vi "To Serial Form.vi"(6 "Serial Version":T1, 10 "Serializer in":refnum<class "Serializer.lvclass">=refnum, 11 "AlicatCommBank in":refnum<class "AlicatCommBank.lvclass">=refnum) -> (0 "error out":errorcluster, 2 "Serializer out":refnum<class "Serializer.lvclass">, 3 "AlicatCommBank out":refnum<class "AlicatCommBank.lvclass">)   [LabVIEW 2014]
uses:
  <userlib>/Serialization/Serializable/Insert Serializable.vi
  <userlib>/Serialization/Serializer/Serializer.lvclass
  <userlib>/Serialization/Serialization Common/Serial Version.ctl
  AlicatCommBank.lvclass
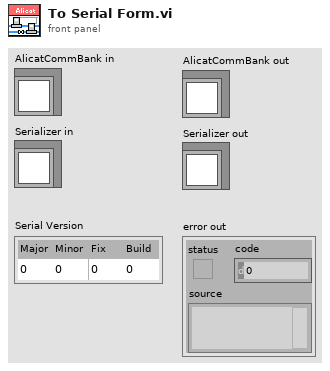
[diagram p1: front panel]
types:
  T1 = typedef "Serialization Common.lvlib/Serial Version.ctl" = cluster{"Major":u16, "Minor":u16, "Fix":u16, "Build":u16}
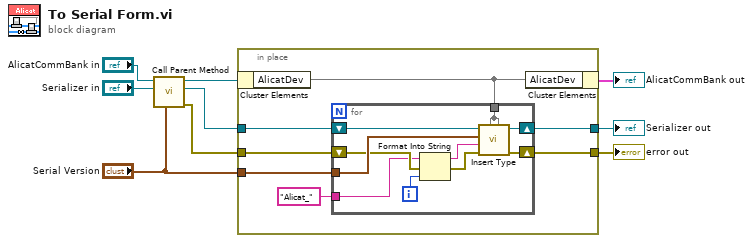
[diagram p0: block diagram]
diagram:
  n1 = call-parent "Call Parent Method"("Serial Version"="Serial Version", "Serializer in"="Serializer in", "Serial IO in"="AlicatCommBank in") -> ("error out"=w4:errorcluster, "Serializer out"=w6:refnum<class "Serializer.lvclass">, "Serial IO out"=w7:refnum<class "AlicatCommBank.lvclass">)  [unwired: 6 in]
  n2 = in-place {
    in-place-border: w6 -> [w16]
    in-place-border: "Serial Version" -> [w15]
    in-place-border: w4 -> [w14]
    in-place-border: [w13] -> w3
    in-place-border: [w11] -> w1
    n3 = in-place-cluster #1(w7) -> ("AlicatDev"=w12)
    n4 = for {
      tunnel: w12 -> [w25]
      tunnel: w15 -> [w24]
      shift-right: [w19] -> w11
      shift-left: w14 -> [w23]
      shift-right: [w18] -> w13
      shift-left: w16 -> [w26]
      tunnel: "Alicat_" ("initial string") -> [w17]
      i -> [w22]
      n5 = Format Into String(initial string=w17, error in=w23, w22) -> (resulting string=w20:string, error out=w21:errorcluster)  [unwired: 1 in]
      n6 = call-poly <userlib>:"Insert Type.vi"("Serializable"=w25, "Default Value"=w25, "error in (no error)"=w21, "Name"=w20, "Serial Version"=w24, "Serializer in"=w26) -> ("error out"=w19:errorcluster, "Serializer out"=w18:refnum<class "Serializer.lvclass">)  [unwired: 4 in]
    }
    n7 = in-place-cluster #1("AlicatDev"=w12) -> (→"AlicatCommBank out":cluster{})
  }
  "error out" <- w1
  "Serializer out" <- w3
